vi "Get Port and line.vi"(10 "PXIXSlotY":string="PXI1Slot5/", 11 "portX/lineY":string="port0/line0") -> (3 "PXI Port Line":tag)   [LabVIEW 2023, in "SPI.lvlib"]
uses:
  SPI.lvlib
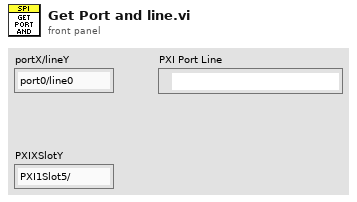
[diagram p1: front panel]
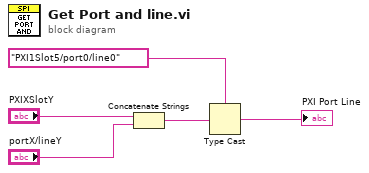
[diagram p0: block diagram]
diagram:
  n1 = Concatenate Strings("PXIXSlotY", "portX/lineY") -> (w3:string)
  n2 = Type Cast(type=tag "PXI1Slot5/port0/line0" ("lines"), x=w3) -> (*(type *) &x=→"PXI Port Line":tag)
